vi "Write Integration ON.vi"(8 "error in (no error)":errorcluster, 10 "Integration ON":bool, 11 "Yokogawa WT2X0 in":refnum<class "Yokogawa WT2X0.lvclass">) -> (0 "error out":errorcluster, 3 "Yokogawa WT2X0 out":refnum<class "Yokogawa WT2X0.lvclass">)   [LabVIEW 2013, in "Universal Power Meter.lvlib" / "Yokogawa WT2X0.lvlib" / "Yokogawa WT2X0.lvclass"]
uses:
  Yokogawa WT2X0.lvclass
  Yokogawa WT2X0.lvclass/Yokogawa WT2X0.ctl
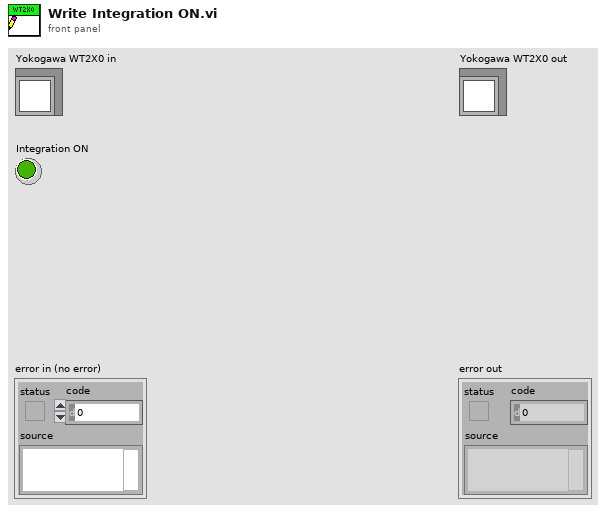
[diagram p1: front panel]
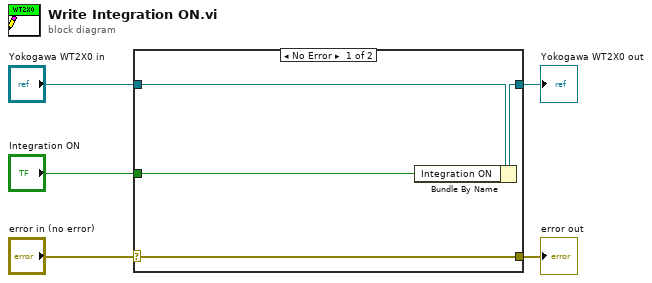
[diagram p0: block diagram]
diagram:
  n1 = case shown="No Error" "error in (no error)" {
    selector: "error in (no error)" -> [w9 w10]
    tunnel: [w9 w10] -> w4
    tunnel: [w7 w11] -> w2
    tunnel: "Yokogawa WT2X0 in" -> [w8 w11]
    tunnel: "Integration ON" -> [w6 _]
    frame No Error {
      n2 = Bundle By Name(cluster=w8, "Integration ON"=w6) -> (w7:refnum<class "Yokogawa WT2X0.lvclass">)
    }
    frame Error {
    }
  }
  "error out" <- w4
  "Yokogawa WT2X0 out" <- w2
